vi "execute.vi"(8 "error in (no error)":errorcluster caption="错误输入（无错误）", 11 "PluginInterface.lvclass":refnum<class "PluginInterface.lvclass">) -> (0 "error out":errorcluster caption="错误输出", 3 "PluginInterface.lvclass":refnum<class "PluginInterface.lvclass">)   [LabVIEW 2021, in "PluginInterface.lvclass"]
doc: "本VI是为《我和LabVIEW》一书编写的示例。\n关于本书的介绍请参考网页：\nhttp://ruanqizhen.spaces.live.com/blog/cns!5852D4F797C53FB6!4310.entry"
uses:
  PluginInterface.lvclass
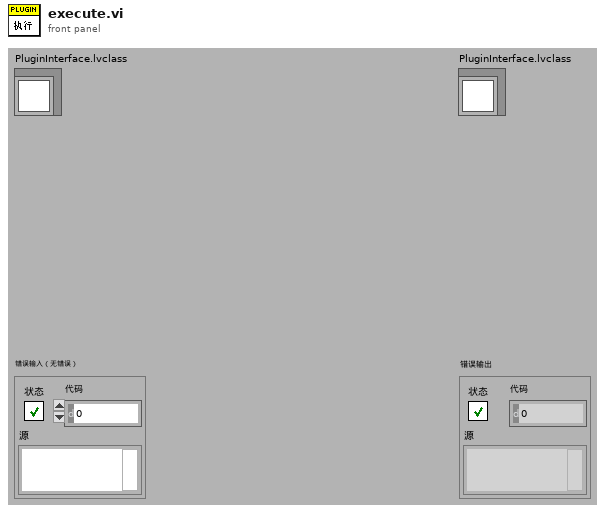
[diagram p1: front panel]
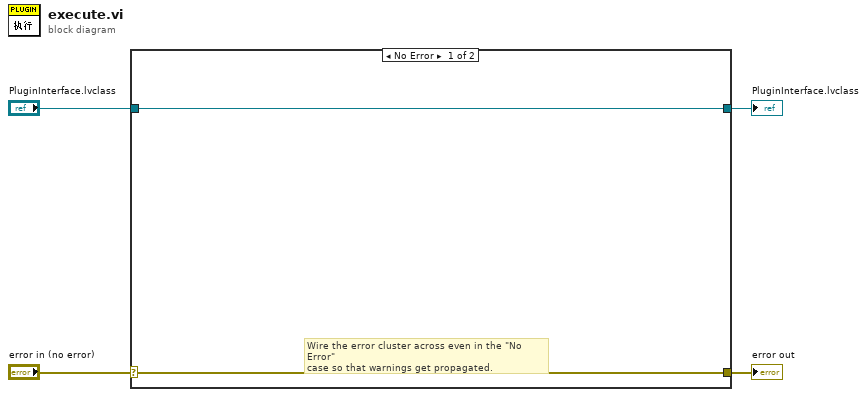
[diagram p0: block diagram]
diagram:
  n1 = case shown="No Error" "error in (no error)" {
    selector: "error in (no error)" -> [w5 w8]
    tunnel: [w5 w8] -> w3
    tunnel: [w6 w7] -> w1
    tunnel: "PluginInterface.lvclass" -> [w6 w7]
    frame No Error {
      # "Wire the error cluster across even in the \"No Error\"\ncase so that warnings get propagated."
    }
    frame Error {
    }
  }
  "error out" <- w3
  "PluginInterface.lvclass" <- w1
